vi "loadInstanceOfEachClassInMemory.vi"() -> (1 "all class names":string[](array[string]), 2 "all classes":refnum<class>[](array[class]))   [LabVIEW 2020, in "JKI JSON Object Serialization.lvlib" / "OOP_Utility.lvlib" / "ClassLoader.lvclass"]
doc: "GCraftsman JSON Object Serialization Toolkit\nwww.GCraftsman.com\nCopyright (c) 2017, GCraftsman"
uses:
  ClassLoader.lvclass
  ClassLoader.lvclass/ClassLoader.ctl
  OOP_Utility.lvlib
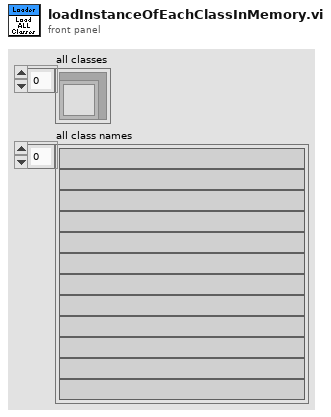
[diagram p1: front panel]
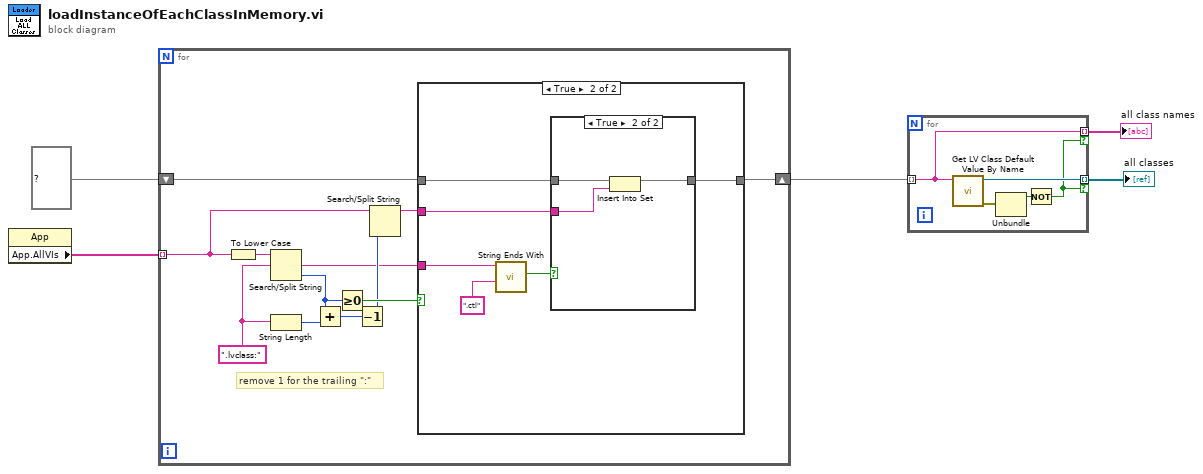
[diagram p0: block diagram]
diagram:
  n1 = property class="App"() -> ("App.AllVIs"=w5:string[])  [unwired: 2 in, 2 out]
  n2 = for {
    tunnel: w5 -> [w10] mode=indexing
    shift-right: [w17] -> w2
    shift-left: set{string} {} ("empty set") -> [w16]
    w15 = ".lvclass:" ("regular expression")
    # "remove 1 for the trailing \":\""
    n3 = To Lower Case(string=w10) -> (all lower case string=w7:string)
    n4 = Search/Split String(string=w7, search string/char (-)=w15) -> (match + rest of string=w6:string, offset of match=w12:i32)  [unwired: 1 in, 1 out]
    n5 = String Length(string=w15) -> (length=w13:i32)
    n6 = Add(x=w12, y=w13) -> (x+y=w11:i32)
    n7 = Greater Or Equal To 0?(x=w12) -> (x >= 0?=w14:bool)
    n8 = Decrement(x=w11) -> (x-1=w9:i32)
    n9 = Search/Split String(string=w10, offset (0)=w9) -> (substring before match=w8:string)  [unwired: 1 in, 2 out]
    n10 = case shown="True" w14 {
      tunnel: [w18 w24] -> w17
      tunnel: w16 -> [w18 w23]
      tunnel: w6 -> [_ w21]
      tunnel: w8 -> [_ w22]
      frame False {
      }
      frame True {
        n11 = call "String Ends With.vi"("ending"=".ctl" ("regular expression"), "string"=w21) -> ("ends with?"=w19:bool)  [unwired: 9 in]
        n12 = case shown="True" w19 {
          tunnel: [w25 w27] -> w24
          tunnel: w23 -> [w25 w28]
          tunnel: w22 -> [_ w26]
          frame False {
          }
          frame True {
            n13 = Insert Into Set(10:w26, 11:w28) -> (3:w27:set{string})  [unwired: 1 out]
          }
        }
      }
    }
  }
  n14 = for {
    tunnel: w2 -> [w30] mode=indexing
    tunnel: [w33] -> w1 mode=indexing if=w29
    tunnel: [w30] -> w4 mode=indexing if=w29
    n15 = call <vilib>:"Get LV Class Default Value By Name.vi"("class name"=w30) -> ("error out"=w32:errorcluster, "object"=w33:refnum<class>)  [unwired: 9 in]
    n16 = Unbundle(w32) -> ("status"=w31:bool)  [unwired: 2 out]
    n17 = Not(x=w31) -> (.not. x?=w29:bool)
  }
  "all classes" <- w1
  "all class names" <- w4
